vi "Initialize Teaching.vi"(7 "# Vectors per Iteration":i64, 8 "Error In":errorcluster, 9 "Validation Set Path In":path, 10 "Teaching Set Path In":path, 11 "Neural Network In":refnum<class "Neural Network.lvclass">) -> (0 "Error Out":errorcluster, 2 "RProp Data":T1, 3 "Neural Network Out":refnum<class "Neural Network.lvclass">)   [LabVIEW 2015, in "Neural Network.lvclass"]
uses:
  Neural Network.lvclass
  Types/2D Array.ctl
  Types/RProp Algorithm.ctl
  Teaching File/Teaching File.lvlib
  Types/Scaling Info.ctl
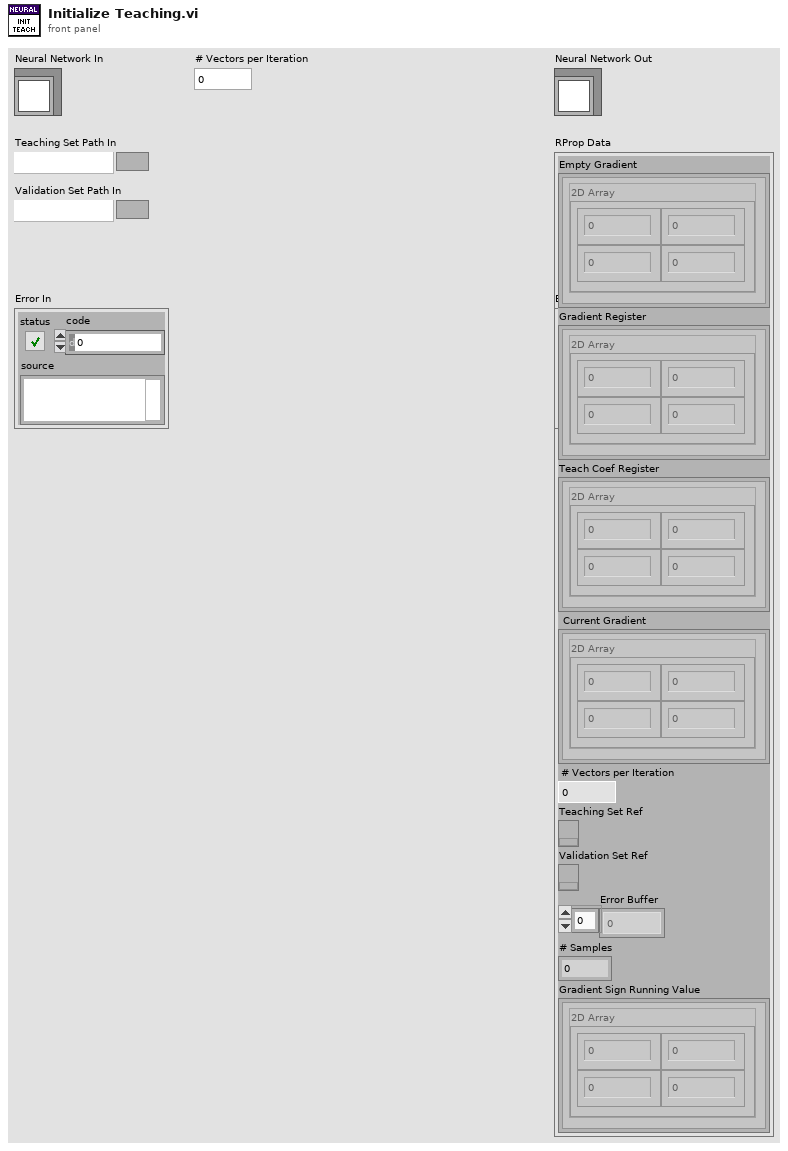
[diagram p1: front panel]
types:
  T1 = typedef "Neural Network.lvclass/RProp Algorithm.ctl" = cluster{"Empty Gradient":T2[], "Gradient Register":T2[], "Teach Coef Register":T2[], "Current Gradient":T2[], "# Vectors per Iteration":i64, "Teaching Set Ref":refnum<k34>, "Validation Set Ref":refnum<k34>, "Error Buffer":dbl[], "# Samples":i64, "Gradient Sign Running Value":T2[]}
  T2 = typedef "Neural Network.lvclass/2D Array.ctl" = cluster{"2D Array":sgl[][]}
  T3 = typedef "Neural Network.lvclass/Scaling Info.ctl" = cluster{"X Scaling Vector":dbl[], "Y Scaling Vector":dbl[]}
  T4 = enum16{"open", "open or create", "create or replace", "create", "open (read-only)"}
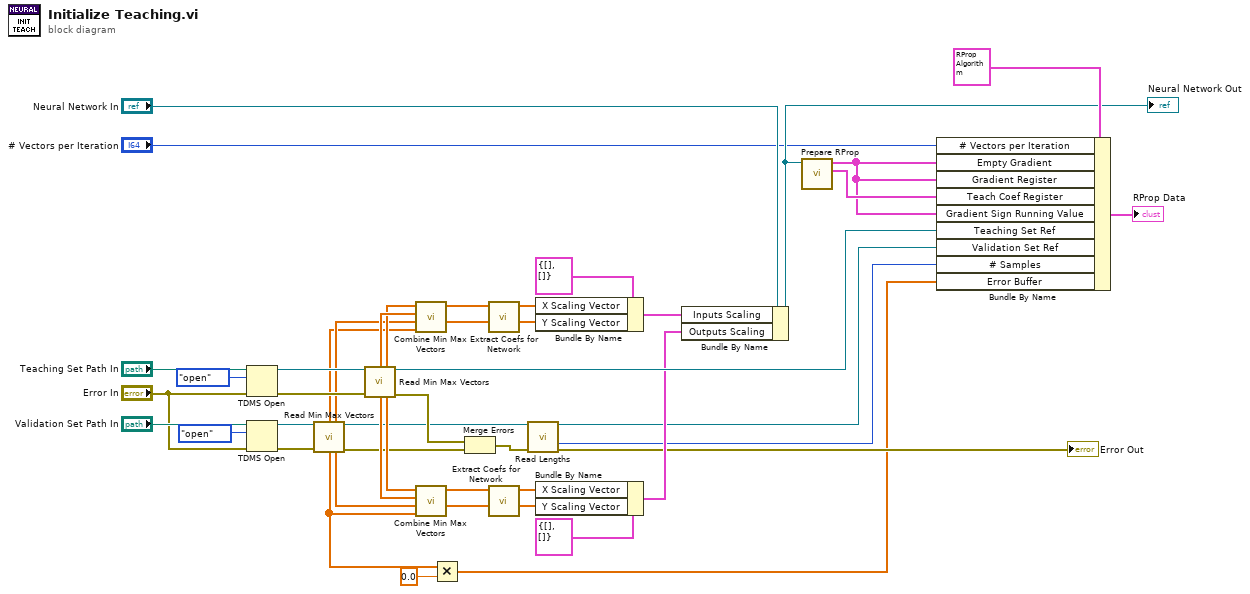
[diagram p0: block diagram]
diagram:
  n1 = TDMS Open(8:"Error In", 10:T4."open" ("operation (0:open)"), 11:"Teaching Set Path In") -> (0:w32:errorcluster, 3:w33:refnum<k34>)  [unwired: 4 in]
  n2 = TDMS Open(8:"Error In", 10:T4."open" ("operation (0:open)"), 11:"Validation Set Path In") -> (0:w30:errorcluster, 3:w31:refnum<k34>)  [unwired: 4 in]
  n3 = call "Read Min Max Vectors.vi"("TDMS In"=w31, "Error In"=w30) -> ("Inputs Min"=w26:dbl[], "Inputs Max"=w27:dbl[], "TDMS Out"=w7:refnum<k34>, "Outputs Min"=w4:dbl[], "Outputs Max"=w18:dbl[], "Error Out"=w15:errorcluster)  [unwired: 8 in]
  n4 = call "Read Min Max Vectors.vi"("TDMS In"=w33, "Error In"=w32) -> ("Inputs Min"=w29:dbl[], "Inputs Max"=w28:dbl[], "TDMS Out"=w35:refnum<k34>, "Outputs Min"=w17:dbl[], "Outputs Max"=w16:dbl[], "Error Out"=w34:errorcluster)  [unwired: 8 in]
  n5 = call "Combine Min Max Vectors.vi"("Other IO Min"=w26, "Other IO Max"=w27, "IO Min"=w29, "IO Max"=w28) -> ("IO Min"=w13:dbl[], "IO Max"=w12:dbl[])  [unwired: 6 in]
  n6 = call "Combine Min Max Vectors.vi"("Other IO Min"=w4, "Other IO Max"=w18, "IO Min"=w17, "IO Max"=w16) -> ("IO Min"=w11:dbl[], "IO Max"=w10:dbl[])  [unwired: 6 in]
  n7 = Multiply(x=w4, y=0.0) -> (x*y=w2:dbl[])
  n8 = Merge Errors(w34, w15) -> (w9:errorcluster)
  n9 = call "Extract Coefs for Network.vi"("Min Array"=w13, "Max Array"=w12) -> ("Y Scaling Vector"=w23:dbl[], "X Scaling Vector"=w24:dbl[])  [unwired: 8 in]
  n10 = call "Extract Coefs for Network.vi"("Min Array"=w11, "Max Array"=w10) -> ("Y Scaling Vector"=w21:dbl[], "X Scaling Vector"=w20:dbl[])  [unwired: 8 in]
  n11 = call "Read Lengths.vi"("TDMS In"=w7, "Error In"=w9) -> ("TDMS Out"=w6:refnum<k34>, "# Samples"=w5:i64, "Error Out"=→"Error Out":errorcluster)  [unwired: 9 in, 2 out]
  n12 = Bundle By Name(cluster=T3 {"X Scaling Vector"=[], "Y Scaling Vector"=[]}, "X Scaling Vector"=w24, "Y Scaling Vector"=w23) -> (w22:T3)
  n13 = Bundle By Name(cluster=T3 {"X Scaling Vector"=[], "Y Scaling Vector"=[]}, "X Scaling Vector"=w20, "Y Scaling Vector"=w21) -> (w14:T3)
  n14 = Bundle By Name(cluster="Neural Network In", "Inputs Scaling"=w22, "Outputs Scaling"=w14) -> (w42:refnum<class "Neural Network.lvclass">)
  "Neural Network Out" <- w42
  n15 = call "Prepare RProp.vi"("Neural Network In"=w42) -> ("Teach Coef Buffer"=w45:T2[], "Gradient Buffer"=w1:T2[])  [unwired: 9 in]
  n16 = Bundle By Name(cluster=T1 {"Empty Gradient"=[], "Gradient Register"=[], "Teach Coef Register"=[], "Current Gradient"=[], "# Vectors per Iteration"=0, "Teaching Set Ref"=refnum, "Validation Set Ref"=refnum, "Error Buffer"=[], "# Samples"=0, "Gradient Sign Running Value"=[]} ("Cluster in"), "# Vectors per Iteration"="# Vectors per Iteration", "Empty Gradient"=w1, "Gradient Register"=w1, "Teach Coef Register"=w45, "Gradient Sign Running Value"=w1, "Teaching Set Ref"=w35, "Validation Set Ref"=w6, "# Samples"=w5, "Error Buffer"=w2) -> (→"RProp Data":T1)
